vi "PRIME Telescope Rd Wr Settings.vi"(8 "error in (no error)":errorcluster, 9 "Name":string, 10 "Write? (F:Read)":bool, 11 "Settings":T1) -> (0 "error out":errorcluster, 3 "Settings":T1)   [LabVIEW 2020]
uses:
  PRIME Telescope cluster Settings.ctl
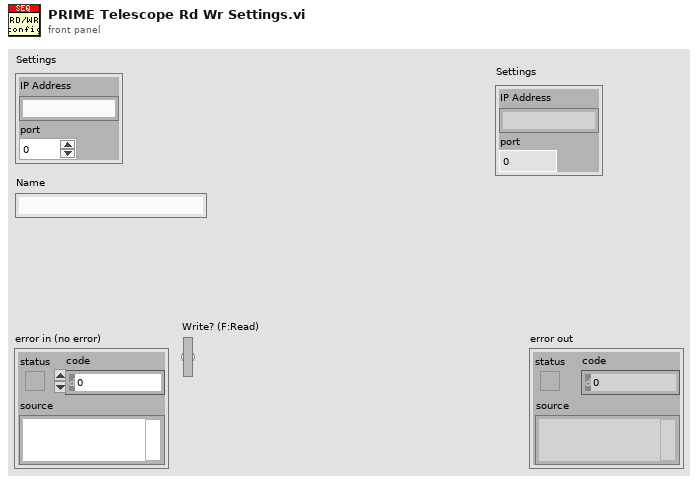
[diagram p1: front panel]
types:
  T1 = typedef "PRIME Telescope cluster Settings.ctl" = cluster{"IP Address":string, "port":u16}
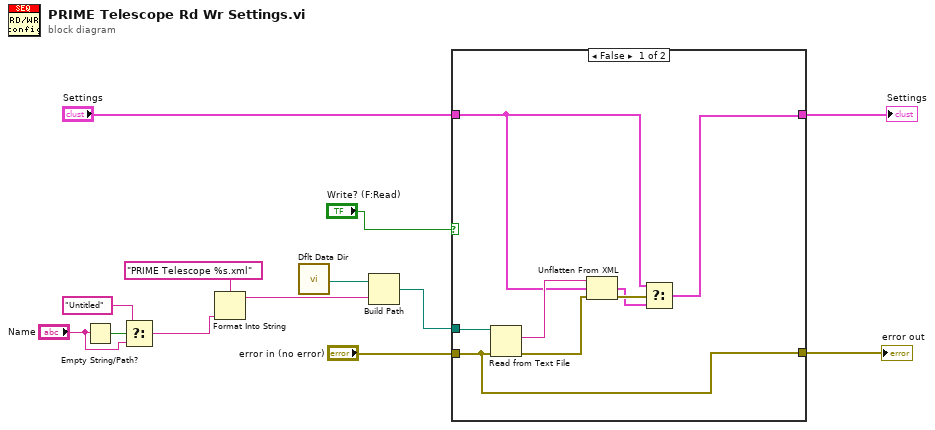
[diagram p0: block diagram]
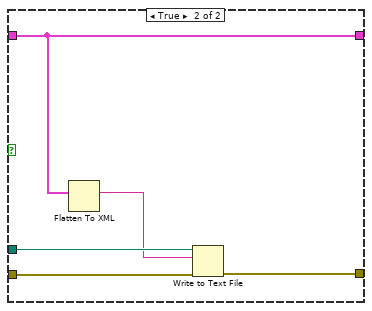
[diagram p2: hidden frame]
diagram:
  n1 = Empty String/Path?(string/path="Name") -> (empty?=w5:bool)
  n2 = Select(t="Untitled", s=w5, f="Name") -> (s? t:f=w2:string)
  n3 = Format Into String(format string="PRIME Telescope %s.xml" ("name or relative path"), w2) -> (resulting string=w1:string)  [unwired: 2 in, 1 out]
  n4 = call <vilib>:"Dflt Data Dir.vi"() -> ("App:Default Data Directory"=w10:path)
  n5 = Build Path(base path=w10, name or relative path=w1) -> (appended path=w9:path)
  n6 = case shown="False" "Write? (F:Read)" {
    tunnel: "error in (no error)" -> [w14 w26]
    tunnel: "Settings" -> [w17 w22]
    tunnel: w9 -> [w21 w25]
    tunnel: [w14 w23] -> w8
    tunnel: [w15 w22] -> w7
    frame False {
      n7 = Read from Text File(file (use dialog)=w21, error in=w14) -> (text=w20:string, error out=w19:errorcluster)  [unwired: 2 in, 2 out]
      n8 = Unflatten From XML(xml string=w20, type=w17, error in (no error)=w19) -> (value=w16:T1, error out=w18:errorcluster)
      n9 = Select(t=w17, s=w18, f=w16) -> (s? t:f=w15:T1)
    }
    frame True {
      n10 = Flatten To XML(6:w22) -> (2:w24:string)
      n11 = Write to Text File(file (use dialog)=w25, text=w24, error in=w26) -> (error out=w23:errorcluster)  [unwired: 1 in, 2 out]
    }
  }
  "error out" <- w8
  "Settings" <- w7
